vi "Read Functional Data (BIN Count).vi"(8 "error in (no error)":errorcluster, 11 "VISA resource name":refnum<visa-resource-name>) -> (0 "error out":errorcluster, 2 "BIN Count Array":i32[](array[numeric]), 3 "VISA resource name out":refnum<visa-resource-name>)   [LabVIEW 2017, in "Agilent E4980.lvlib"]
doc: "Returns the comparator BIN count results. \n\n<B>Notes:</B>\n(1) Elements of the array are: <Bin 1>, <Bin 2>, <Bin 3>, <Bin 4>, <Bin 5>, <Bin 6>, <Bin 7>, <Bin 8>, <Bin 9>, <Out of Bin>, <Aux Bin>."
uses:
  Agilent E4980.lvlib
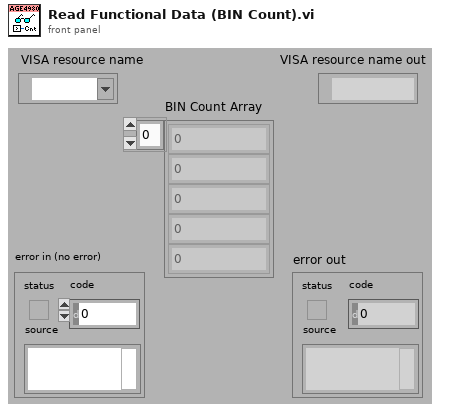
[diagram p1: front panel]
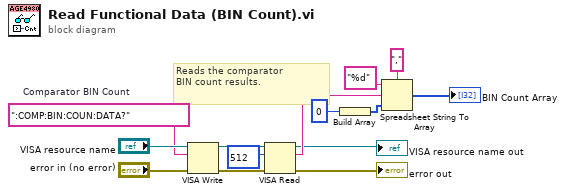
[diagram p0: block diagram]
diagram:
  w12 = ":COMP:BIN:COUN:DATA?"  # Comparator BIN Count
  # "Reads the comparator\nBIN count results."
  n1 = VISA Write(VISA resource name="VISA resource name", write buffer=w12, error in (no error)="error in (no error)") -> (VISA resource name out=w11:refnum<visa-resource-name>, error out=w10:errorcluster)  [unwired: 1 out]
  n2 = VISA Read(VISA resource name=w11, byte count=u32 512, error in (no error)=w10) -> (VISA resource name out=→"VISA resource name out":refnum<visa-resource-name>, read buffer=w4:string, error out=→"error out":errorcluster)  [unwired: 1 out]
  n3 = Build Array(0) -> (w7:i32[])
  n4 = Spreadsheet String To Array(delimiter (Tab)="," ("spreadsheet string"), format string="%d", spreadsheet string=w4, array type (2D Dbl)=w7) -> (array=→"BIN Count Array":i32[])
